vi "Test.vi"() -> ()   [LabVIEW 2023, in "Modbus TCP Micro.lvlib"]
uses:
  Modbus TCP Micro.lvlib
  Read Bool.vi
  Read U16.vi
  Modbus Request.vi
panel:
  out "Discrete Inputs":bool[](array[boolean])
  out "Array 2":u16[](array[numeric])
  out "Array":u16[](array[numeric])
  out "Coil States":bool[](array[boolean])
  out "error out":errorcluster
  in  "error in (no error)":errorcluster
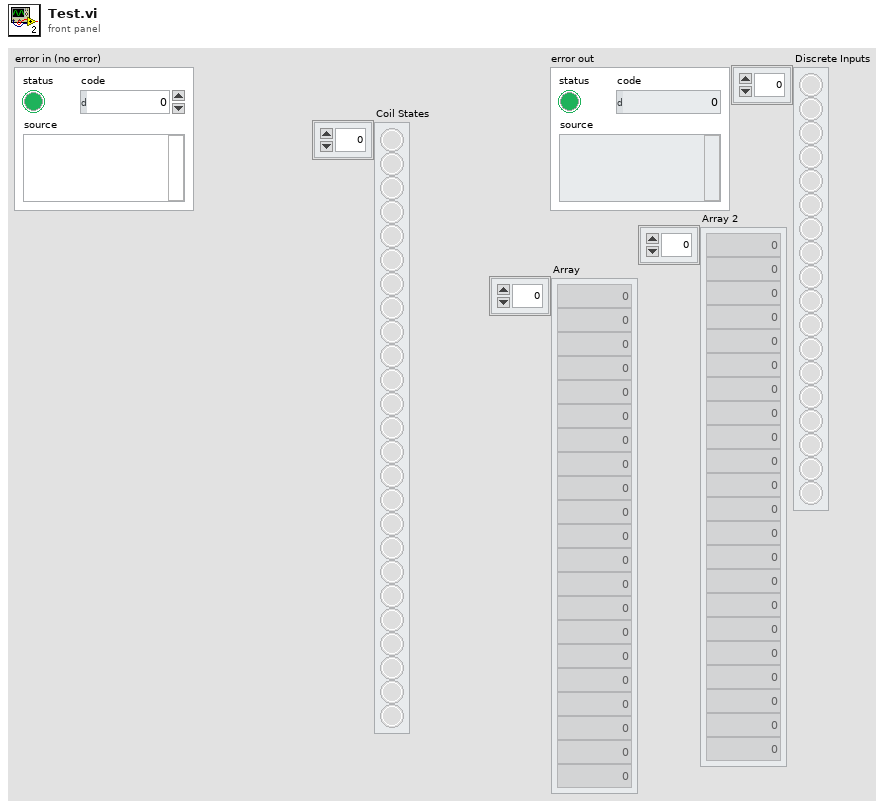
[diagram p1: front panel]
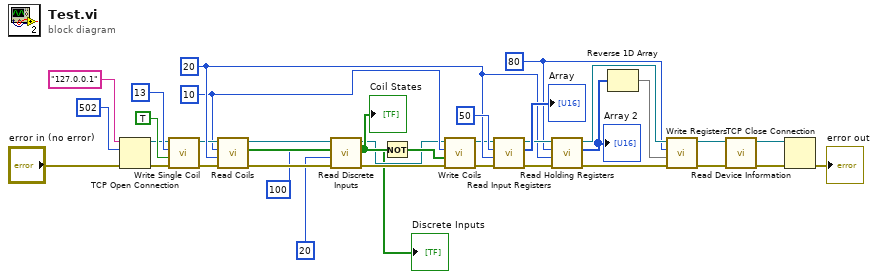
[diagram p0: block diagram]
diagram:
  w18 = u16 80 ("Start Address")
  w22 = u16 20 ("Number of Registers")
  w13 = u16 10 ("Start Address")
  n1 = TCP Open Connection(address="127.0.0.1", remote port or service name=u16 502, error in (no error)="error in (no error)") -> (connection ID=w10:refnum<k5>, error out=w31:errorcluster)  [unwired: 2 in]
  n2 = call "Write Single Coil.vi"("error in (no error)"=w31, "Value"=TRUE, "Address"=u16 13 ("Start Address"), "TCP Network Connection in"=w10) -> ("error out"=w35:errorcluster, "TCP Network Connection out"=w21:refnum<k5>)  [unwired: 6 in]
  n3 = call "Read Coils.vi"("error in (no error)"=w35, "Number of Registers"=w22, "Start Address"=w13, "TCP Network Connection in"=w21) -> ("error out"=w28:errorcluster, "Coil States"=w12:bool[], "TCP Network Connection out"=w8:refnum<k5>)  [unwired: 5 in]
  "Coil States" <- w12
  n4 = call "Read Discrete Inputs.vi"("error in (no error)"=w28, "Number of Registers"=u16 20, "Start Address"=u16 100, "TCP Network Connection in"=w8) -> ("error out"=w9:errorcluster, "Discrete Inputs"=→"Discrete Inputs":bool[], "TCP Network Connection out"=w7:refnum<k5>)  [unwired: 5 in]
  n5 = Not(x=w12) -> (.not. x?=w11:bool[])
  n6 = call "Write Coils.vi"("error in (no error)"=w9, "Value"=w11, "Start Address"=w13, "TCP Network Connection in"=w7) -> ("error out"=w15:errorcluster, "TCP Network Connection out"=w14:refnum<k5>)  [unwired: 6 in]
  n7 = call "Read Input Registers.vi"("error in (no error)"=w15, "Number of Registers"=w22, "Start Address"=u16 50, "TCP Network Connection in"=w14) -> ("error out"=w27:errorcluster, "Array"=→"Array":u16[], "TCP Network Connection out"=w23:refnum<k5>)  [unwired: 5 in]
  n8 = call "Read Holding Registers.vi"("error in (no error)"=w27, "Number of Registers"=w22, "Start Address"=w18, "TCP Network Connection in"=w23) -> ("error out"=w24:errorcluster, "Array"=w17:u16[], "TCP Network Connection out"=w19:refnum<k5>)  [unwired: 5 in]
  "Array 2" <- w17
  n9 = Reverse 1D Array(array=w17) -> (reversed array=w16:u16[])
  n10 = call "Write Registers.vi"("error in (no error)"=w24, "Values"=w16, "Start Address"=w18, "TCP Network Connection in"=w19) -> ("error out"=w20:errorcluster, "TCP Network Connection out"=w2:refnum<k5>)  [unwired: 6 in]
  n11 = call "Read Device Information.vi"("error in (no error)"=w20, "TCP Network Connection in"=w2) -> ("error in (no error) 2"=w3:errorcluster, "TCP Network Connection out"=w1:refnum<k5>)  [unwired: 7 in, 1 out]
  n12 = TCP Close Connection(connection ID=w1, error in (no error)=w3) -> (error out=→"error out":errorcluster)  [unwired: 1 in, 1 out]
